vi "DriveReadEncoder.vi"(8 "error in":errorcluster, 11 "ModualNamePrefix":i32) -> (0 "error out":errorcluster, 2 "SWERVE_DRIVE_MODULE_POSITION":T1={"Distance"=0.0, "Angle"={"VALUE"=0.0, "COS"=1.0, "SIN"=0.0}, "P"=FALSE} {"Angle"."SIN" format="%13.4f"; "Angle"."COS" format="%13.4f"; "Angle"."VALUE" format="%13.4f"}, 3 "SWERVE_DRIVE_MODULE_STATE":T3={"Speed"=0.0, "Angle"={"VALUE"=0.0, "COS"=1.0, "SIN"=0.0}} {"Angle"."SIN" format="%13.4f"; "Angle"."COS" format="%13.4f"; "Angle"."VALUE" format="%13.4f"})   [LabVIEW 2023]
uses:
  <vilib>/Rock Robotics/Network Tables/NT Write Number.vi
  <vilib>/Rock Robotics/WPI/ThirdParty/JAS_Junk/TrajLib/Trajectory_Library.lvlib
  DriveGlobal.vi
  <vilib>/Rock Robotics/WPI/ThirdParty/REV Robotics/REVLib/SubVI/Public/SPARK Get Encoder Status Position.vi
  <vilib>/Rock Robotics/WPI/ThirdParty/REV Robotics/REVLib/SubVI/Public/SPARK Get Encoder Status Velocity.vi
  <vilib>/Rock Robotics/WPI/ThirdParty/Phoenix6/getters/GetCANcoder_Velocity.vi
  <vilib>/Rock Robotics/WPI/ThirdParty/Phoenix6/getters/GetCANcoder_Position.vi
  <vilib>/Rock Robotics/WPI/ThirdParty/Phoenix6/getters/GetCANcoder_AbsPosition.vi
  <vilib>/Rock Robotics/WPI/ThirdParty/JAS_Junk/TrajLib/TypeDef/ROTATION2D.ctl
  <vilib>/Rock Robotics/WPI/ThirdParty/JAS_Junk/TrajLib/TypeDef/SWERVE_DRIVE_MODULE_STATE.ctl
  <vilib>/Rock Robotics/WPI/ThirdParty/JAS_Junk/TrajLib/TypeDef/SWERVE_DRIVE_MODULE_POSITION.ctl
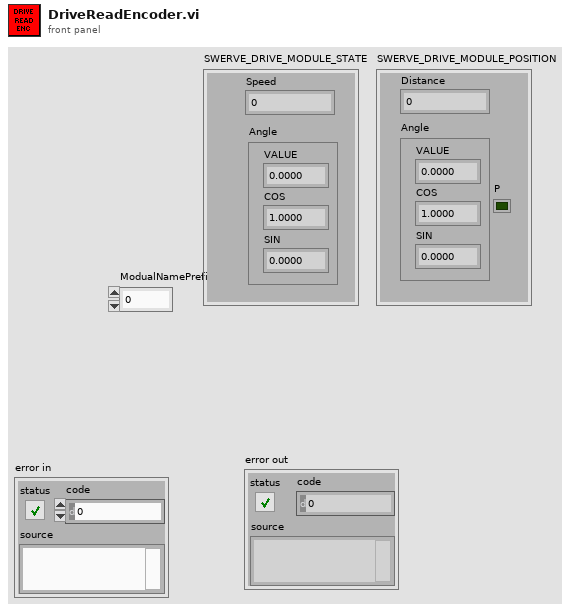
[diagram p1: front panel]
types:
  T1 = typedef "Trajectory_Library.lvlib/SWERVE_DRIVE_MODULE_POSITION.ctl" = cluster{"Distance":dbl, "Angle":T2, "P":bool}
  T2 = typedef "Trajectory_Library.lvlib/ROTATION2D.ctl" = cluster{"VALUE":dbl, "COS":dbl, "SIN":dbl}
  T3 = typedef "Trajectory_Library.lvlib/SWERVE_DRIVE_MODULE_STATE.ctl" = cluster{"Speed":dbl, "Angle":T2}
  T4 = typedef "WPI_MotorControlDeviceRef.ctl" = cluster{"DeviceStatus":errorcluster, "Type":T5, "PWM":cluster{"PWM Channel":T6, "DeadBand":T7}, "CAN":cluster{"Device Number":u8, "SetOutput VI Ref":variant, "GetOutput VI Ref":variant, "Enable VI Ref":variant, "Disable VI Ref":variant, "Data":variant}, "Invert":bool, "DIO PWM":cluster{"PWM \"Enable\" Channel":T6, "DIOChannel":T8, "PWM Rate":dbl}}
  T5 = typedef "WPI_MotorControlType.ctl" = enum16{"PWM", "CAN", "DIO PWM"}
  T6 = typedef "FPGA_DIOPWMChannel.ctl" = enum8{"PWM 0", "PWM 1", "PWM 2", "PWM 3", "PWM 4", "PWM 5", "PWM 6", "PWM 7", "PWM 8", "PWM 9", "PWM MXP 0", "PWM MXP 1", "PWM MXP 2", "PWM MXP 3", "PWM MXP 4", "PWM MXP 5", "PWM MXP 6", "PWM MXP 7", "PWM MXP 8", "PWM MXP 9", "Invalid"}
  T7 = typedef "WPI_PWMDeadband.ctl" = cluster{"Name":string, "maxPositivePwm":i32, "minPositivePwm":i32, "centerPwm":i32, "maxNegativePwm":i32, "minNegativePwm":i32, "angularRange":u16}
  T8 = typedef "FPGA_DIOChannel.ctl" = enum8{"DIO 0", "DIO 1", "DIO 2", "DIO 3", "DIO 4", "DIO 5", "DIO 6", "DIO 7", "DIO 8", "DIO 9", "DIO MXP 0", "DIO MXP 1", "DIO MXP 2", "DIO MXP 3", "DIO MXP 4", "DIO MXP 5", "DIO MXP 6", "DIO MXP 7", "DIO MXP 8", "DIO MXP 9", "DIO MXP 10", "DIO MXP 11", "DIO MXP 12", "DIO MXP 13", "DIO MXP 14", "DIO MXP 15", "SPI Port CS1", "SPI Port CS2", "SPI Port CS3", "SPI Port MISO", "SPI Port MOSI", "Invalid"}
  T9 = typedef "DeviceReference.ctl" = cluster{"CANbus Name":string, "Device Encoding":u32, "Device Name":string}
  T10 = cluster{"Value":dbl, "System Timestamp":dbl, "CANivore Timestamp":dbl, "ECU Timestamp":dbl}
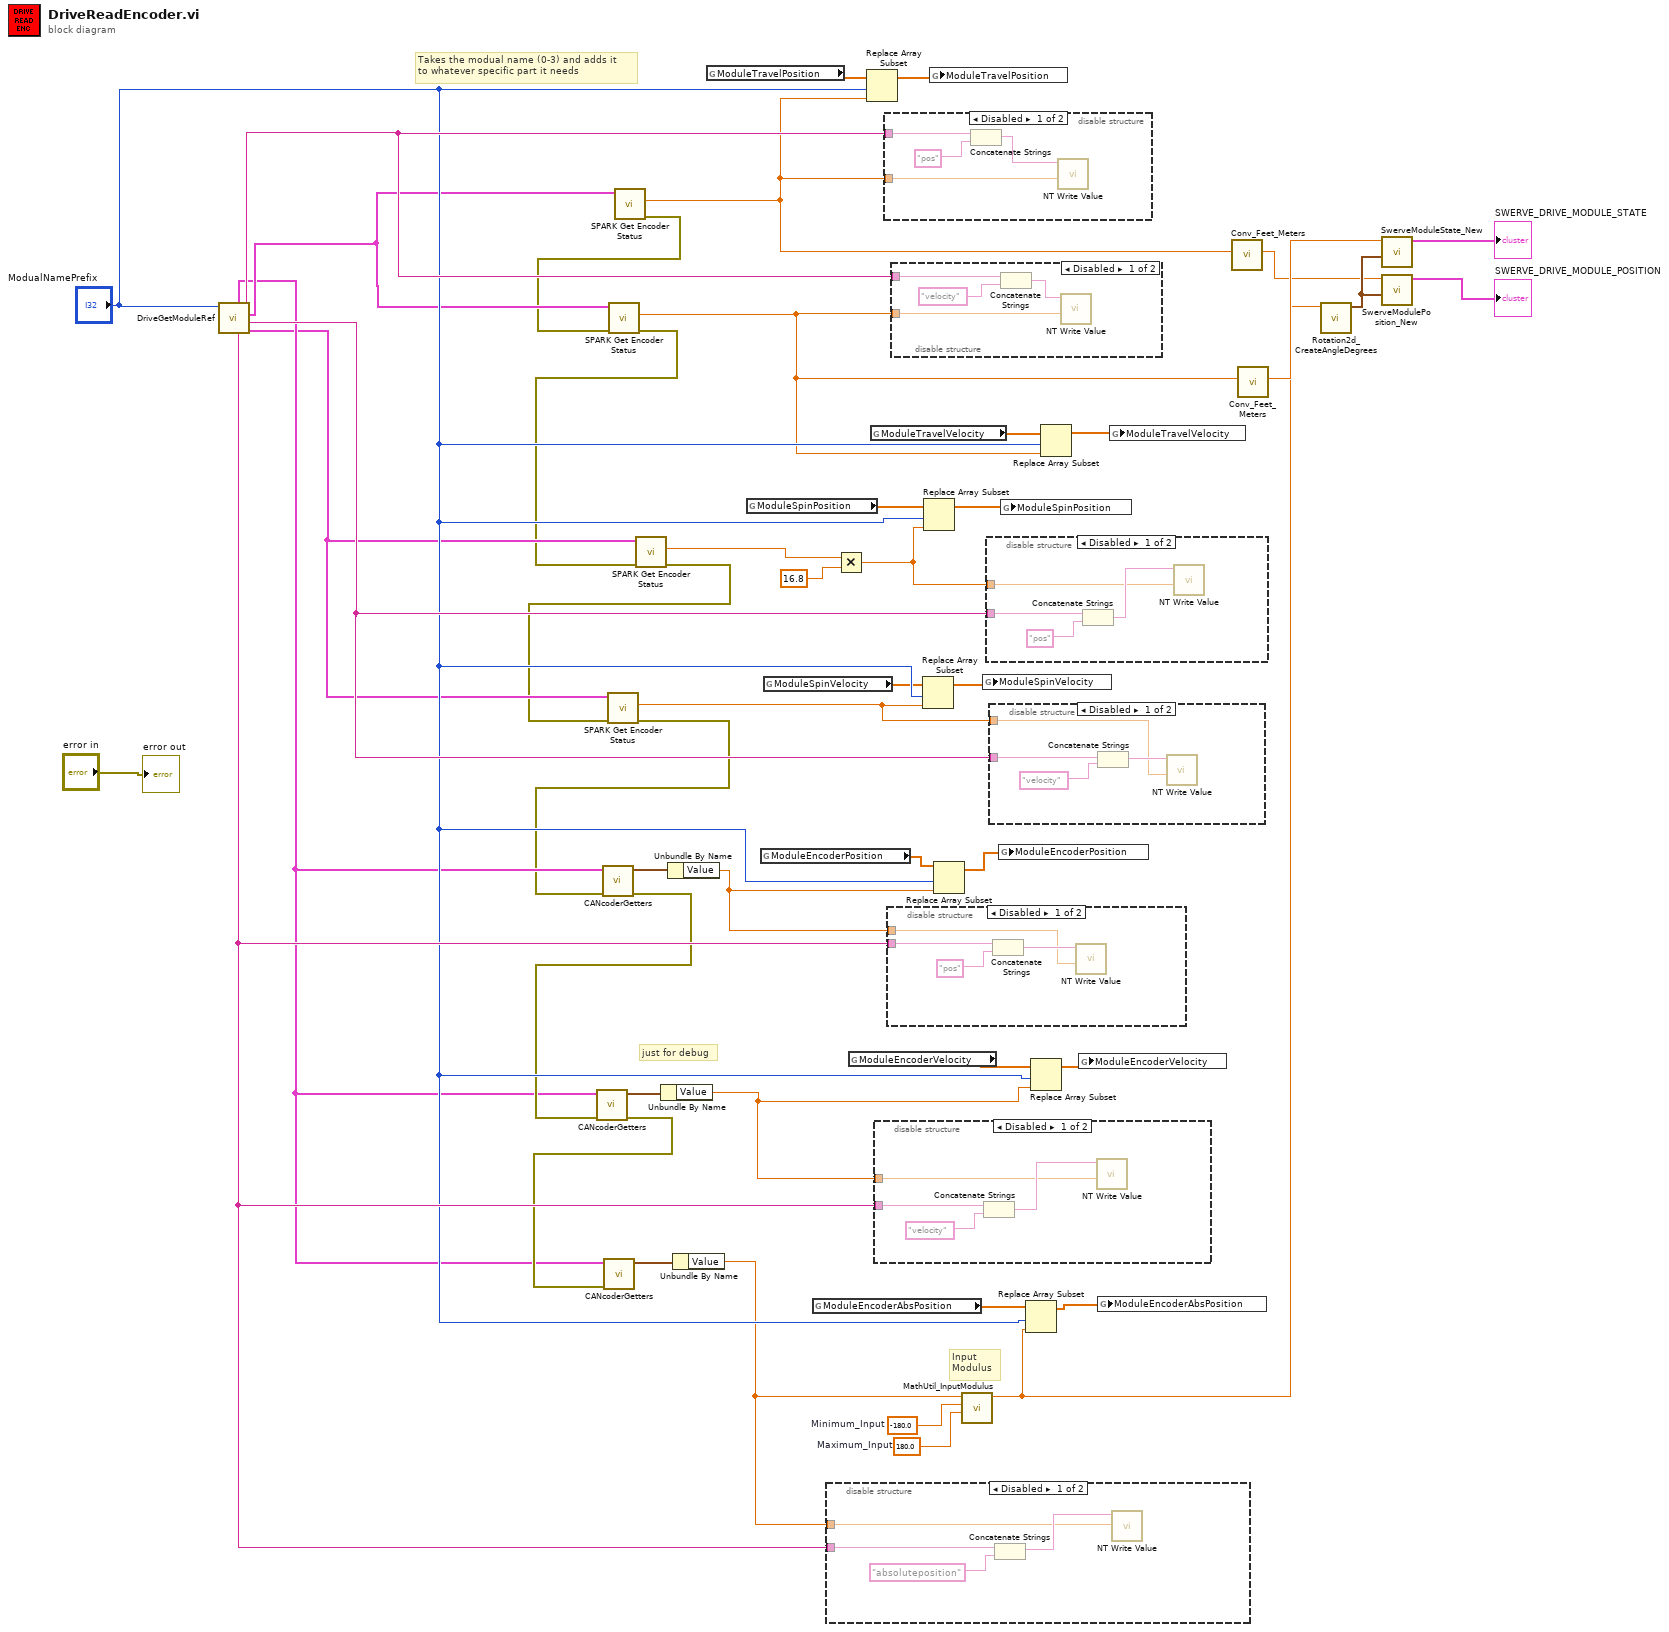
[diagram p0: block diagram]
diagram:
  w44 = -180.0  # Minimum_Input
  w43 = 180.0  # Maximum_Input
  # "Input\nModulus"
  # "just for debug"
  # "Takes the modual name (0-3) and adds it \nto whatever specific part it needs"
  n1 = call "DriveGetModuleRef.vi"("ModualNamePrefix"="ModualNamePrefix") -> ("SpinMot"=w5:T4, "SpinStr"=w38:string, "TravMot"=w24:T4, "TravStr"=w37:string, "EncStr"=w36:string, "AbsEncoder"=w15:T9)  [unwired: 5 in]
  n2 = call-poly <vilib>:"SPARK Get Encoder Status.vi"("MotorControlDevRef in"=w24) -> ("error out"=w23:errorcluster, "Sensor Position"=w25:dbl)  [unwired: 7 in, 2 out]
  n3 = call-poly <vilib>:"SPARK Get Encoder Status.vi"("error in (no error)"=w23, "MotorControlDevRef in"=w24) -> ("error out"=w3:errorcluster, "Sensor Velocity"=w22:dbl)  [unwired: 6 in, 2 out]
  n4 = call-poly <vilib>:"SPARK Get Encoder Status.vi"("error in (no error)"=w3, "MotorControlDevRef in"=w5) -> ("error out"=w2:errorcluster, "Sensor Position"=w6:dbl)  [unwired: 6 in, 2 out]
  n5 = call-poly <vilib>:"SPARK Get Encoder Status.vi"("error in (no error)"=w2, "MotorControlDevRef in"=w5) -> ("error out"=w1:errorcluster, "Sensor Velocity"=w4:dbl)  [unwired: 6 in, 2 out]
  n6 = call-poly <vilib>:"CANcoderGetters.vi"("error in"=w1, "DeviceReference"=w15) -> ("error out"=w19:errorcluster, "Output"=w21:T10)  [unwired: 8 in]
  n7 = call-poly <vilib>:"CANcoderGetters.vi"("error in"=w19, "DeviceReference"=w15) -> ("error out"=w16:errorcluster, "Output"=w18:T10)  [unwired: 8 in]
  n8 = call-poly <vilib>:"CANcoderGetters.vi"("error in"=w16, "DeviceReference"=w15) -> ("Output"=w8:T10)  [unwired: 8 in, 1 out]
  n9 = Unbundle By Name(w18) -> ("Value"=w17:dbl)
  n10 = Unbundle By Name(w21) -> ("Value"=w20:dbl)
  n11 = Unbundle By Name(w8) -> ("Value"=w7:dbl)
  n12 = global read "DriveGlobal.vi" "ModuleTravelPosition"() -> (w40:dbl[])
  n13 = global read "DriveGlobal.vi" "ModuleSpinPosition"() -> (w13:dbl[])
  n14 = global read "DriveGlobal.vi" "ModuleEncoderPosition"() -> (w33:dbl[])
  n15 = global read "DriveGlobal.vi" "ModuleSpinVelocity"() -> (w10:dbl[])
  n16 = global read "DriveGlobal.vi" "ModuleEncoderAbsPosition"() -> (w29:dbl[])
  n17 = disable-structure shown="Disabled" {
    disable-tunnel: w36 -> [w50 _]
    disable-tunnel: w7 -> [w49 _]
    frame Disabled {
      n18 = Concatenate Strings(w50, "absoluteposition" ("refnum name")) -> (w51:string)
      n19 = call-poly <vilib>:"NT Write Value.vi"("value"=w49, "name"=w51) -> ()  [unwired: 9 in, 1 out]
    }
    frame Enabled {
    }
  }
  n20 = Multiply(x=w6, y=16.8) -> (x*y=w11:dbl)
  n21 = global read "DriveGlobal.vi" "ModuleEncoderVelocity"() -> (w31:dbl[])
  n22 = Replace Array Subset(array=w40, new element=w25, index="ModualNamePrefix") -> (w39:dbl[])
  n23 = global read "DriveGlobal.vi" "ModuleTravelVelocity"() -> (w35:dbl[])
  n24 = disable-structure shown="Disabled" {
    disable-tunnel: w36 -> [w54 _]
    disable-tunnel: w17 -> [w53 _]
    frame Disabled {
      n25 = Concatenate Strings(w54, "velocity" ("refnum name")) -> (w55:string)
      n26 = call-poly <vilib>:"NT Write Value.vi"("value"=w53, "name"=w55) -> ()  [unwired: 9 in, 1 out]
    }
    frame Enabled {
    }
  }
  n27 = disable-structure shown="Disabled" {
    disable-tunnel: w37 -> [w58 _]
    disable-tunnel: w25 -> [w57 _]
    frame Disabled {
      n28 = Concatenate Strings(w58, "pos" ("refnum name")) -> (w59:string)
      n29 = call-poly <vilib>:"NT Write Value.vi"("value"=w57, "name"=w59) -> ()  [unwired: 9 in, 1 out]
    }
    frame Enabled {
    }
  }
  n30 = disable-structure shown="Disabled" {
    disable-tunnel: w36 -> [w62 _]
    disable-tunnel: w20 -> [w61 _]
    frame Disabled {
      n31 = Concatenate Strings(w62, "pos" ("refnum name")) -> (w63:string)
      n32 = call-poly <vilib>:"NT Write Value.vi"("value"=w61, "name"=w63) -> ()  [unwired: 9 in, 1 out]
    }
    frame Enabled {
    }
  }
  n33 = disable-structure shown="Disabled" {
    disable-tunnel: w37 -> [w66 _]
    disable-tunnel: w22 -> [w65 _]
    frame Disabled {
      n34 = Concatenate Strings(w66, "velocity" ("refnum name")) -> (w67:string)
      n35 = call-poly <vilib>:"NT Write Value.vi"("value"=w65, "name"=w67) -> ()  [unwired: 9 in, 1 out]
    }
    frame Enabled {
    }
  }
  n36 = Replace Array Subset(array=w10, new element=w4, index="ModualNamePrefix") -> (w9:dbl[])
  n37 = Replace Array Subset(array=w13, new element=w11, index="ModualNamePrefix") -> (w12:dbl[])
  n38 = global write "DriveGlobal.vi" "ModuleTravelPosition"(w39) -> ()
  n39 = Replace Array Subset(array=w33, new element=w20, index="ModualNamePrefix") -> (w32:dbl[])
  n40 = call <vilib>:"MathUtil_InputModulus.vi"("Maximum_Input"=w43, "Minimum_Input"=w44, "Input"=w7) -> ("modulus"=w26:dbl)  [unwired: 8 in]
  n41 = global write "DriveGlobal.vi" "ModuleSpinVelocity"(w9) -> ()
  n42 = disable-structure shown="Disabled" {
    disable-tunnel: w38 -> [w72 _]
    disable-tunnel: w11 -> [w69 _]
    frame Disabled {
      n43 = Concatenate Strings(w72, "pos" ("refnum name")) -> (w70:string)
      n44 = call-poly <vilib>:"NT Write Value.vi"("value"=w69, "name"=w70) -> ()  [unwired: 9 in, 1 out]
    }
    frame Enabled {
    }
  }
  n45 = disable-structure shown="Disabled" {
    disable-tunnel: w38 -> [w76 _]
    disable-tunnel: w4 -> [w73 _]
    frame Disabled {
      n46 = Concatenate Strings(w76, "velocity" ("refnum name")) -> (w74:string)
      n47 = call-poly <vilib>:"NT Write Value.vi"("value"=w73, "name"=w74) -> ()  [unwired: 9 in, 1 out]
    }
    frame Enabled {
    }
  }
  n48 = global write "DriveGlobal.vi" "ModuleEncoderPosition"(w32) -> ()
  n49 = global write "DriveGlobal.vi" "ModuleSpinPosition"(w12) -> ()
  n50 = Replace Array Subset(array=w29, new element=w26, index="ModualNamePrefix") -> (w28:dbl[])
  n51 = Replace Array Subset(array=w31, new element=w17, index="ModualNamePrefix") -> (w30:dbl[])
  n52 = Replace Array Subset(array=w35, new element=w22, index="ModualNamePrefix") -> (w34:dbl[])
  n53 = global write "DriveGlobal.vi" "ModuleEncoderVelocity"(w30) -> ()
  n54 = global write "DriveGlobal.vi" "ModuleEncoderAbsPosition"(w28) -> ()
  n55 = global write "DriveGlobal.vi" "ModuleTravelVelocity"(w34) -> ()
  n56 = call <vilib>:"Conv_Feet_Meters.vi"("Feet"=w25) -> ("Meters"=w41:dbl)  [unwired: 10 in]
  n57 = call <vilib>:"Conv_Feet_Meters.vi"("Feet"=w22) -> ("Meters"=w42:dbl)  [unwired: 10 in]
  n58 = call <vilib>:"Rotation2d_CreateAngleDegrees.vi"("Angle_Degrees"=w26) -> ("ROTATION"=w47:T2)  [unwired: 10 in]
  n59 = call <vilib>:"SwerveModuleState_New.vi"("ROTATION"=w47, "Speed"=w42) -> ("SWERVE_DRIVE_MODULE_STATE"=→"SWERVE_DRIVE_MODULE_STATE":T3)  [unwired: 9 in]
  n60 = call <vilib>:"SwerveModulePosition_New.vi"("ROTATION"=w47, "Distance"=w41) -> ("SWERVE_DRIVE_MODULE_POSITION"=→"SWERVE_DRIVE_MODULE_POSITION":T1)  [unwired: 9 in]
  "error out" <- "error in"
